vi "DSF.Shared.Configuration.Framework.Convert.To JSON Cluster.vi"(8 "error in (no error)":errorcluster, 11 "Framework Configuration in":refnum<class "DSF.Shared.Configuration.Framework.lvclass">) -> (0 "error out":errorcluster, 2 "Framework Config (JSON)":T1, 3 "Framework Configuration out":refnum<class "DSF.Shared.Configuration.Framework.lvclass">)   [LabVIEW 2017, in "DSF.Shared.lvlib" / "DSF.Shared.Configuration.Framework.lvclass"]
uses:
  DSF.Shared.Configuration.Framework.lvclass
  Typedefs/DSF.Shared.Refactor.Typedefs.Framework Configuration.Aggregate.JSON.ctl
  Typedefs/DSF.Shared.Refactor.Typedefs.Plugin Configuration.Aggregate.JSON.ctl
  Typedefs/DSF.Shared.Typedefs.Cycle Timing Factors.ctl
  Typedefs/DSF.Shared.Refactor.Typedefs.Transfer Group Configuration.Aggregate.JSON.ctl
  Typedefs/DSF.Shared.Refactor.Typedefs.JSON.Transfer Configuration.ctl
  Typedefs/DSF.Shared.Refactor.Typedefs.JSON.Channel Array Configuration.ctl
  DSF.Shared.Configuration.Framework.lvclass/DSF.Shared.Configuration.Framework.ctl
  DSF.Shared.lvlib
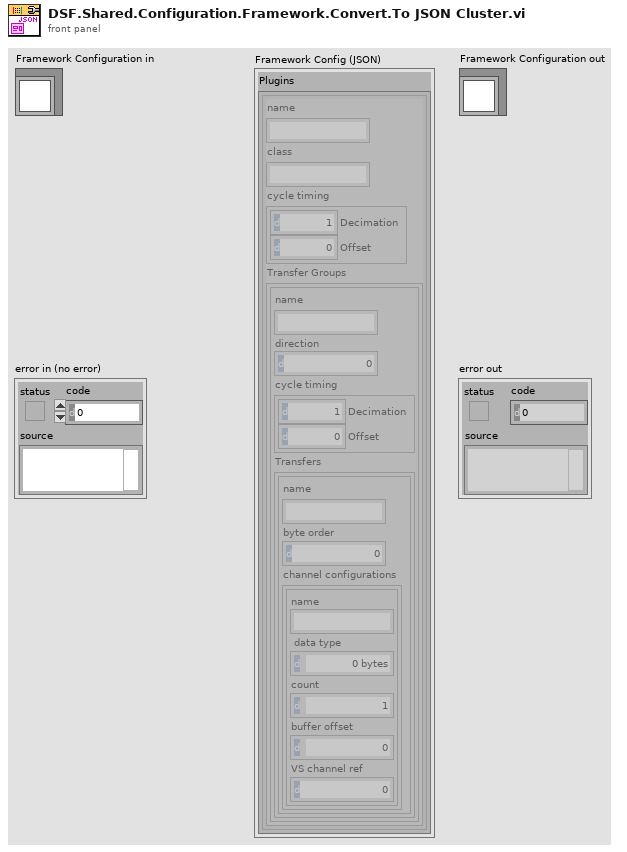
[diagram p1: front panel]
types:
  T1 = typedef "DSF.Shared.lvlib/DSF.Shared.Refactor.Typedefs.Framework Configuration.Aggregate.JSON.ctl" = cluster{"Plugins":T2[]}
  T2 = typedef "DSF.Shared.lvlib/DSF.Shared.Refactor.Typedefs.Plugin Configuration.Aggregate.JSON.ctl" = cluster{"name":string, "class":string, "cycle timing":T3, "Transfer Groups":T4[]}
  T3 = typedef "DSF.Shared.lvlib/DSF.Shared.Typedefs.Cycle Timing Factors.ctl" = cluster{"Decimation":u64, "Offset":u64}
  T4 = typedef "DSF.Shared.lvlib/DSF.Shared.Refactor.Typedefs.Transfer Group Configuration.Aggregate.JSON.ctl" = cluster{"name":string, "direction":u8, "cycle timing":T3, "Transfers":T5[]}
  T5 = typedef "DSF.Shared.lvlib/DSF.Shared.Refactor.Typedefs.JSON.Transfer Configuration.ctl" = cluster{"name":string, "byte order":u8, "channel configurations":T6[]}
  T6 = typedef "DSF.Shared.lvlib/DSF.Shared.Refactor.Typedefs.JSON.Channel Array Configuration.ctl" = cluster{"name":string, "data type":u8, "count":u64, "buffer offset":u64, "VS channel ref":u64}
  T7 = typedef "DSF.Shared.lvlib/DSF.Shared.Refactor.Typedefs.Framework Configuration.Aggregate.ctl" = cluster{"Plugins":T8[]}
  T8 = typedef "DSF.Shared.lvlib/DSF.Shared.Refactor.Typedefs.Plugin Configuration.Aggregate.ctl" = cluster{"name":string, "class":string, "cycle timing":T3, "Transfer Groups":T9[]}
  T9 = typedef "DSF.Shared.lvlib/DSF.Shared.Refactor.Typedefs.Transfer Group Configuration.Aggregate.ctl" = cluster{"name":string, "direction":T10, "cycle timing":T3, "Transfers":T11[]}
  T10 = typedef "DSF.Shared.lvlib/DSF.Shared.Typedefs.Direction.ctl" = enum8{"Tx", "Rx"}
  T11 = typedef "DSF.Shared.lvlib/DSF.Shared.Refactor.Typedefs.Transfer Configuration.ctl" = cluster{"name":string, "byte order":T12, "channel configurations":T13[]}
  T12 = typedef "DSF.Shared.lvlib/DSF.Shared.Typedefs.Byte Order.ctl" = enum8{"big-endian", "little-endian"}
  T13 = typedef "DSF.Shared.lvlib/DSF.Shared.Refactor.Typedefs.Channel Array Configuration.ctl" = cluster{"name":string, "data type":T14, "count":u64, "buffer offset":u64, "engine offset":u64}
  T14 = typedef "DSF.Shared.lvlib/DSF.Shared.Typedefs.Data Type.ctl" = enum8{"Bool", "SGL", "DBL", "I8", "I16", "I32", "I64", "U8", "U16", "U32", "U64"}
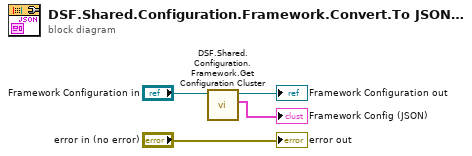
[diagram p0: block diagram]
diagram:
  n1 = call "DSF.Shared.Configuration.Framework.Get Configuration Cluster.vi"("Framework Configuration in"="Framework Configuration in") -> ("Framework Configuration"=→"Framework Config (JSON)":T7, "Framework Configuration out"=→"Framework Configuration out":refnum<class "DSF.Shared.Configuration.Framework.lvclass">)  [unwired: 9 in]
  "error out" <- "error in (no error)"
